vi "ADIS16448_RoboRIO_Teensy_Loop.vi"(8 "error in":errorcluster, 11 "SerialPortRefIn":T1) -> ()   [LabVIEW 2016, in "ADIS16448-Teensy.lvlib"]
uses:
  ADIS16448-Teensy.lvlib
  <vilib>/Rock Robotics/WPI/SerialPort/WPI_SerialPortRef.ctl
  Util_Functions.ctl
panel:
  in  "Main Name":string
  out "Parsed Serial Data":dbl[](array[numeric])
  out "Raw Serial Data":string
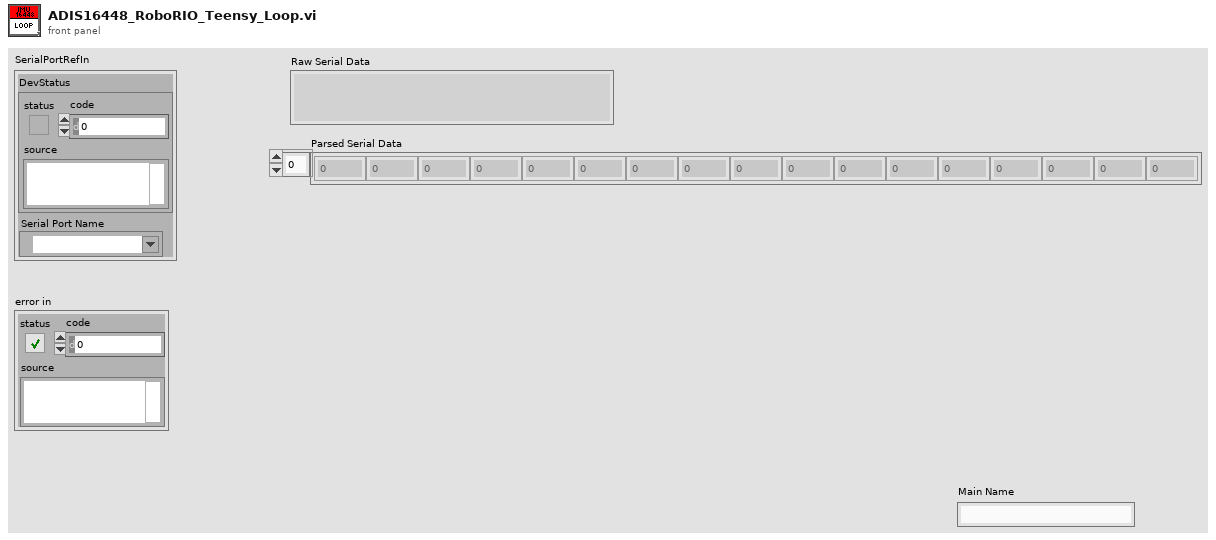
[diagram p1: front panel]
types:
  T1 = typedef "WPI_SerialPortRef.ctl" = cluster{"DevStatus":errorcluster, "Serial Port Name":refnum<visa-resource-name>}
  T2 = cluster{"X Gyro":dbl, "Y Gyro":dbl, "Z Gyro":dbl, "X Accel":dbl, "Y Accel":dbl, "Z Acel":dbl, "X Mag":dbl, "Y Mag":dbl, "Z Mag":dbl, "Baro":dbl, "Temp":dbl}
  T3 = enum16{"set", "get", "set reset", "set function"}
  T4 = cluster{"X Angle":dbl, "Y Angle":dbl, "Z Angle":dbl}
  T5 = typedef "Util_Functions.ctl" = enum16{"None", "Calibrate"}
  T6 = enum32{"Bad", "Idle", "Run top level", "Running"}
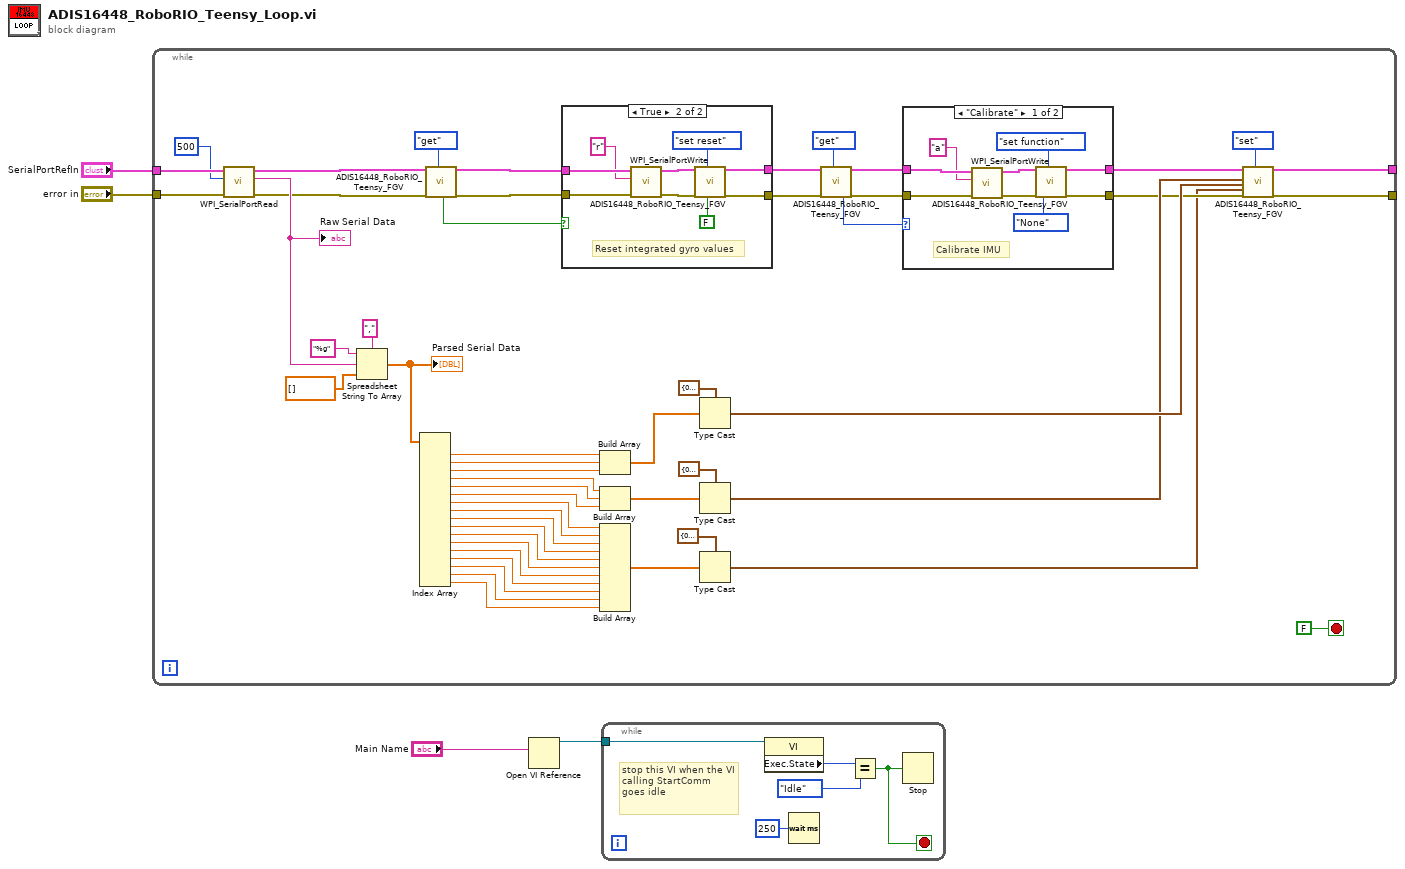
[diagram p0: block diagram]
diagram:
  n1 = while {
    tunnel: "SerialPortRefIn" -> [w56]
    tunnel: "error in" -> [w55]
    tunnel: [w42] -> _
    tunnel: [w41] -> _
    stop <- FALSE stop-if-true
    n2 = call <vilib>:"WPI_SerialPortRead.vi"("error in (no error)"=w55, "Num Bytes to Read"=u32 500, "SerialPortRef"=w56) -> ("error out"=w43:errorcluster, "Buffer"=w50:string, "SerialPortRef"=w47:T1)  [unwired: 6 in]
    "Raw Serial Data" <- w50
    n3 = Spreadsheet String To Array(delimiter (Tab)="," ("delimiter"), format string="%g", spreadsheet string=w50, array type (2D Dbl)=dbl[] []) -> (array=w39:dbl[])
    "Parsed Serial Data" <- w39
    n4 = Index Array(array=w39) -> (element #1=w38:dbl, element #2=w37:dbl, element #3=w36:dbl, element #4=w34:dbl, element #5=w33:dbl, element #6=w32:dbl, element #7=w25:dbl, element #8=w24:dbl, element #9=w26:dbl, element #10=w14:dbl, element #11=w13:dbl, element #12=w12:dbl, element #13=w11:dbl, element #14=w10:dbl, element #15=w9:dbl, element #16=w8:dbl, element #17=w7:dbl)  [unwired: 17 in]
    n5 = call "ADIS16448_RoboRIO_Teensy_FGV.vi"("SerialPortRefIn"=w47, "error in"=w43, "Operation"=enum16{"set", "get", "set reset"}."get") -> ("Reset Out"=w46:bool, "SerialPortRefOut"=w45:T1, "error out"=w44:errorcluster)  [unwired: 10 in, 4 out]
    n6 = case shown="True" w46 {
      tunnel: w45 -> [w69 w78]
      tunnel: w44 -> [w68 w77]
      tunnel: [w69 w73] -> w22
      tunnel: [w68 w72] -> w19
      frame False {
      }
      frame True {
        # "Reset integrated gyro values"
        n7 = call <vilib>:"WPI_SerialPortWrite.vi"("error in (no error)"=w77, "Buffer"="r", "SerialPortRef"=w78) -> ("error out"=w71:errorcluster, "SerialPortRef"=w70:T1)  [unwired: 6 in, 1 out]
        n8 = call "ADIS16448_RoboRIO_Teensy_FGV.vi"("SerialPortRefIn"=w70, "error in"=w71, "Operation"=enum16{"set", "get", "set reset"}."set reset", "Reset"=FALSE) -> ("SerialPortRefOut"=w73:T1, "error out"=w72:errorcluster)  [unwired: 9 in, 5 out]
      }
    }
    n9 = Build Array(w38, w37, w36) -> (w35:dbl[])
    n10 = Build Array(w34, w33, w32) -> (w31:dbl[])
    n11 = Build Array(w25, w24, w26, w14, w13, w12, w11, w10, w9, w8, w7) -> (w23:dbl[])
    n12 = Type Cast(type=cluster{"Pitch":dbl, "Roll":dbl, "Yaw":dbl} {"Pitch"=0.0, "Roll"=0.0, "Yaw"=0.0} ("IMU AHRS"), x=w35) -> (*(type *) &x=w28:cluster{"Pitch":dbl, "Roll":dbl, "Yaw":dbl})
    n13 = Type Cast(type=T4 {"X Angle"=0.0, "Y Angle"=0.0, "Z Angle"=0.0} ("IMU Angles"), x=w31) -> (*(type *) &x=w27:T4)
    n14 = Type Cast(type=T2 {"X Gyro"=0.0, "Y Gyro"=0.0, "Z Gyro"=0.0, "X Accel"=0.0, "Y Accel"=0.0, "Z Acel"=0.0, "X Mag"=0.0, "Y Mag"=0.0, "Z Mag"=0.0, "Baro"=0.0, "Temp"=0.0} ("IMU Instant"), x=w23) -> (*(type *) &x=w5:T2)
    n15 = call "ADIS16448_RoboRIO_Teensy_FGV.vi"("SerialPortRefIn"=w22, "error in"=w19, "Operation"=T3."get") -> ("Function Out"=w17:T5, "SerialPortRefOut"=w21:T1, "error out"=w20:errorcluster)  [unwired: 10 in, 4 out]
    n16 = case shown="\"Calibrate\"" w17 {
      tunnel: w21 -> [w65 w67]
      tunnel: w20 -> [w64 w66]
      tunnel: [w62 w67] -> w16
      tunnel: [w61 w66] -> w15
      frame "Calibrate" {
        # "Calibrate IMU"
        n17 = call <vilib>:"WPI_SerialPortWrite.vi"("error in (no error)"=w64, "Buffer"="a", "SerialPortRef"=w65) -> ("error out"=w60:errorcluster, "SerialPortRef"=w59:T1)  [unwired: 6 in, 1 out]
        n18 = call "ADIS16448_RoboRIO_Teensy_FGV.vi"("SerialPortRefIn"=w59, "error in"=w60, "Function"=Util_Functions."None", "Operation"=T3."set function") -> ("SerialPortRefOut"=w62:T1, "error out"=w61:errorcluster)  [unwired: 9 in, 5 out]
      }
      frame "None", Default {
      }
    }
    n19 = call "ADIS16448_RoboRIO_Teensy_FGV.vi"("SerialPortRefIn"=w16, "IMU Angles"=w27, "IMU AHRS"=w28, "IMU Instant"=w5, "error in"=w15, "Operation"=enum16{"set", "get", "set reset"}."set") -> ("SerialPortRefOut"=w42:T1, "error out"=w41:errorcluster)  [unwired: 7 in, 5 out]
  }
  n20 = Open VI Reference(vi path="Main Name") -> (vi reference=w2:refnum<vi>)  [unwired: 1 in, 5 out]
  n21 = while {
    tunnel: w2 -> [w80]
    stop <- w79 stop-if-true
    # "stop this VI when the VI calling StartComm goes idle"
    n22 = property class="VI"(reference=w80) -> ("Exec.State"=w82:T6)  [unwired: 1 in, 2 out]
    n23 = Wait (ms)(milliseconds to wait=u32 250) -> ()  [unwired: 1 out]
    n24 = Equal?(x=w82, y=T6."Idle" ("Execution:State")) -> (x = y?=w79:bool)
    n25 = Stop(stop? (T)=w79) -> ()
  }
